vi "initialize.vi"(4 "Tolerance (m)":dbl, 5 "Timeout (s)":dbl=-1.0, 6 "Duration (s)":dbl=-1.0, 7 "error in (no error)":errorcluster, 8 "Points of Interest":T2[](array[typedef]) {"North" format="%#_10f"; "East" format="%#_8f"}, 9 "Mission Type":T1, 10 "Idle in":refnum<class "Idle.lvclass">) -> (0 "error out":errorcluster, 3 "Idle out":refnum<class "Idle.lvclass">)   [LabVIEW 2012, in "Idle.lvclass"]
uses:
  Idle.lvclass
  Data/TypeDefs/UTM Location.ctl
  Data/TypeDefs/MissionTypeControl.ctl
  Idle.lvclass/Idle.ctl
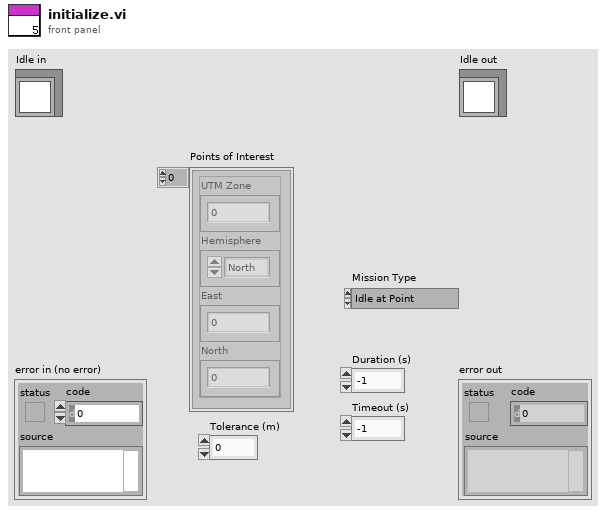
[diagram p1: front panel]
types:
  T1 = typedef "MissionTypeControl.ctl" = enum16{"Idle at Point", "Drive to Waypoint", "Round Buoy to Port", "Round Buoy to Starboard", "Pass Between Buoys", "Station Keeping"}
  T2 = typedef "UTM Location.ctl" = cluster{"UTM Zone":dbl, "Hemisphere":enum16{"North", "South"}, "East":dbl, "North":dbl}
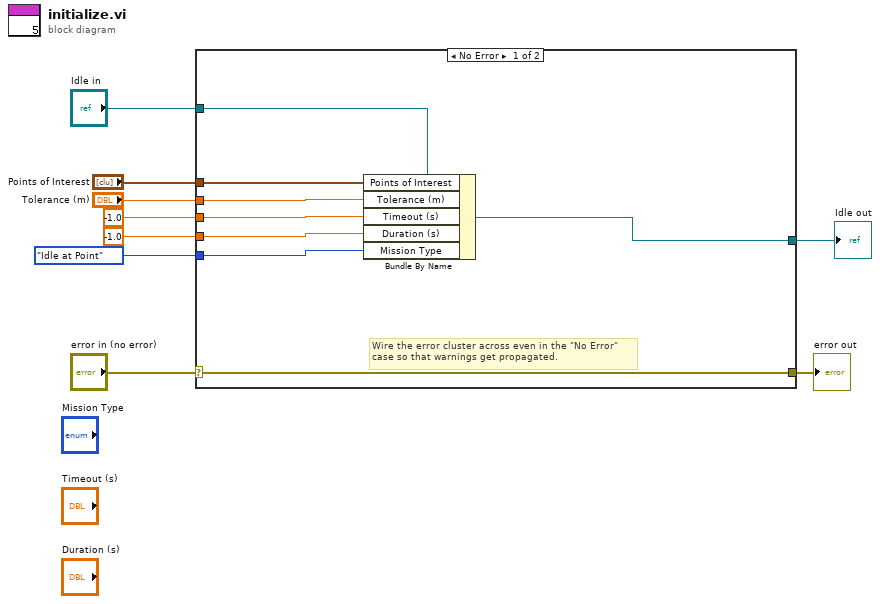
[diagram p0: block diagram]
diagram:
  n1 = case shown="No Error" "error in (no error)" {
    selector: "error in (no error)" -> [w17 w19]
    tunnel: [w17 w19] -> w8
    tunnel: [w10 w18] -> w6
    tunnel: "Idle in" -> [w16 w18]
    tunnel: "Points of Interest" -> [w15 _]
    tunnel: "Tolerance (m)" -> [w14 _]
    tunnel: -1.0 ("Timeout (s)") -> [w13 _]
    tunnel: -1.0 ("Duration (s)") -> [w12 _]
    tunnel: MissionTypeControl."Idle at Point" ("Mission Type") -> [w11 _]
    frame No Error {
      # "Wire the error cluster across even in the \"No Error\"\ncase so that warnings get propagated."
      n2 = Bundle By Name(cluster=w16, "Points of Interest"=w15, "Tolerance (m)"=w14, "Timeout (s)"=w13, "Duration (s)"=w12, "Mission Type"=w11) -> (w10:refnum<class "Idle.lvclass">)
    }
    frame Error {
    }
  }
  "error out" <- w8
  "Idle out" <- w6
